vi "OC2 Read Buffer.vi"(5 "COMS IN":bool, 8 "error in (no error)":errorcluster, 9 "fedback read buffer":string, 11 "VISA resource name":refnum<visa-resource-name>) -> (0 "error out":errorcluster, 1 "Report string":string, 2 "RX packet ok":bool, 3 "VISA resource name out":refnum<visa-resource-name>, 4 "feedback buffer":string)   [LabVIEW 2009]
panel:
  out "return count":u32
  # "Read buffer"
  # "j520.004;0.002;4;4;100.151;100.151;100.000;100.000;1;1;16"
  # "V1.02"
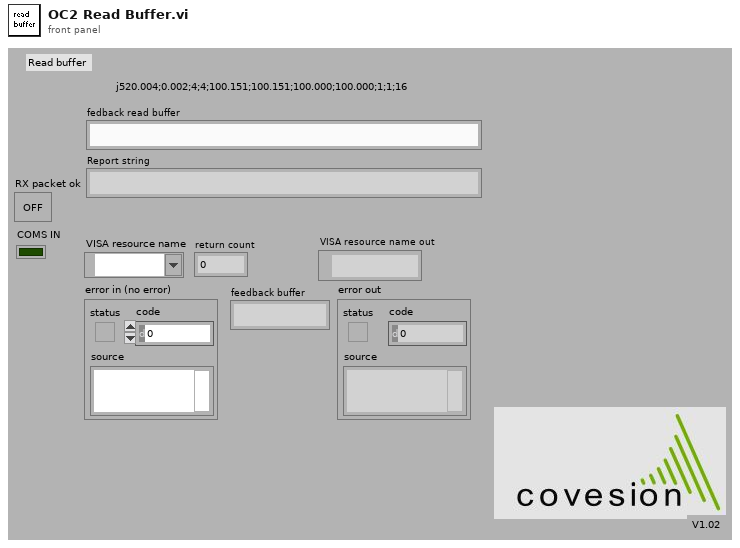
[diagram p1: front panel]
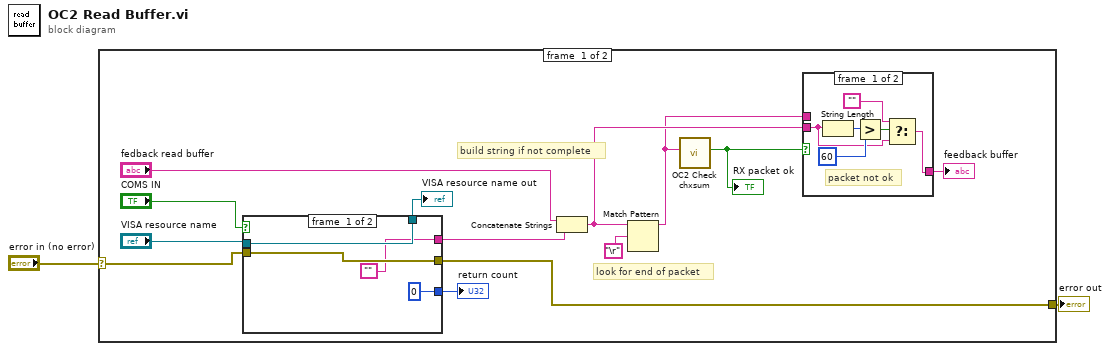
[diagram p0: block diagram]
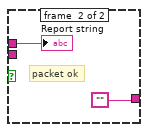
[diagram p2: hidden frame]
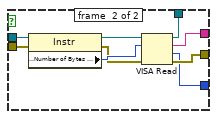
[diagram p3: hidden frame]
diagram:
  n1 = case shown="No Error" "error in (no error)" {
    selector: "error in (no error)" -> [w3 w37]
    tunnel: [w6 w37] -> w2
    frame #0 {
      # "look for end of packet"
      # "build string if not complete"
      n2 = case shown="True" "COMS IN" {
        tunnel: ["" ("Empty String Constant") w35] -> w10
        tunnel: "VISA resource name" -> [w27 w34]
        tunnel: w3 -> [w26 w33]
        tunnel: [w27 w31] -> w7
        tunnel: [w26 w30] -> w6
        tunnel: [u32 0 ("return count") w28] -> w13
        frame #0 {
        }
        frame #1 {
          n3 = property on="Property Node" class="Instr"(reference=w34, error in=w33) -> (reference out=w29:refnum<visa-resource-name>, error out=w32:errorcluster, "Serial Settings:Number of Bytes at Serial Port"=w36:u32)
          n4 = VISA Read(VISA resource name=w29, byte count=w36, error in (no error)=w32) -> (VISA resource name out=w31:refnum<visa-resource-name>, read buffer=w35:string, return count=w28:u32, error out=w30:errorcluster)
        }
      }
      "return count" <- w13
      "VISA resource name out" <- w7
      n5 = Concatenate Strings("fedback read buffer", w10) -> (w8:string)
      n6 = Match Pattern(string=w8, regular expression="\r" ("format string")) -> (before substring=w5:string)  [unwired: 1 in, 3 out]
      n7 = call "OC2 Check chxsum.vi"("report string"=w5) -> ("RX packet ok"=w4:bool)  [unwired: 10 in]
      "RX packet ok" <- w4
      n8 = case shown="True" w4 {
        tunnel: w8 -> [w18 _]
        tunnel: [w16 "" ("Empty String Constant")] -> w11
        tunnel: w5 -> [_ w22]
        frame #0 {
          # "packet not ok"
          n9 = String Length(string=w18) -> (length=w21:i32)
          n10 = Greater?(x=w21, y=60) -> (0:w19:bool)
          n11 = Select(t="" ("Empty String Constant"), s=w19, f=w18) -> (s? t:f=w16:string)
        }
        frame #1 {
          # "packet ok"
          "Report string" <- w22
        }
      }
      "feedback buffer" <- w11
    }
    frame #1 {
    }
  }
  "error out" <- w2
